vi "PropertyNodes.vi"() -> ()   [LabVIEW 2015]
panel:
  in  "stop":bool
  in  "Colors [4] 2":cluster{u32, u32}[](array[cluster])
  out "Colors [4]":cluster{u32, u32}[](array[cluster])
  in  "Legend:Visible":bool
  in  "Y Scale.Range:Maximum":dbl
  in  "Y Scale.Range:Minimum":dbl
  in  "X Scale.Range:Maximum":dbl
  in  "X Scale.Range:Minimum":dbl
  in  "Disabled 2":T1(ring)
  out "Waveform Chart":dbl(graph)
  in  "Numeric 2":dbl
  in  "Boolean 2":bool
  in  "Boolean":bool
  in  "Disabled":T1(ring)
  in  "Numeric":dbl
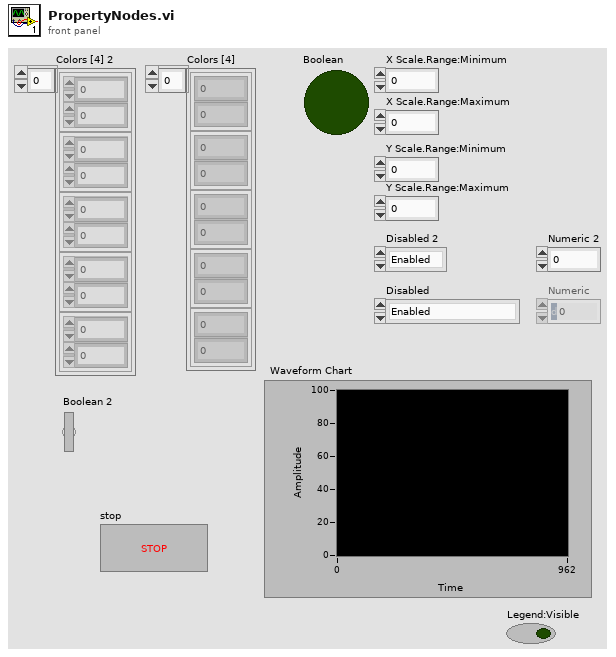
[diagram p1: front panel]
types:
  T1 = enum8{"Enabled", "Disabled", "Disabled and Grayed Out"}
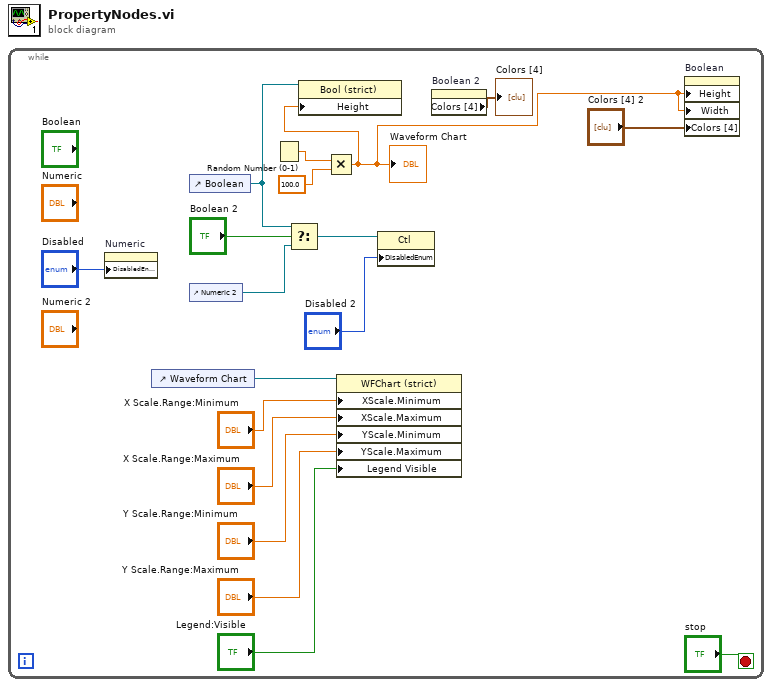
[diagram p0: block diagram]
diagram:
  n1 = while {
    stop <- "stop" stop-if-true
    n2 = property on="Numeric" class="DigNum (strict)"("DisabledEnum"="Disabled") -> ()  [unwired: 2 in, 2 out]
    n3 = control-ref of="Waveform Chart"() -> (w12:refnum<vi>)
    n4 = control-ref of="Boolean"() -> (w17:refnum<vi>)
    n5 = control-ref of="Numeric 2"() -> (w13:refnum<vi>)
    n6 = Random Number (0-1)() -> (number: 0 to 1=w14:dbl)
    n7 = Select(t=w17, s="Boolean 2", f=w13) -> (s? t:f=w2:refnum<vi>)
    n8 = Multiply(x=w14, y=100.0) -> (x*y=w4:dbl)
    "Waveform Chart" <- w4
    n9 = property class="Bool (strict)"(reference=w17, "Height"=w4) -> ()  [unwired: 1 in, 2 out]
    n10 = property class="WFChart (strict)"(reference=w12, "XScale.Minimum"="X Scale.Range:Minimum", "XScale.Maximum"="X Scale.Range:Maximum", "YScale.Minimum"="Y Scale.Range:Minimum", "YScale.Maximum"="Y Scale.Range:Maximum", "Legend Visible"="Legend:Visible") -> ()  [unwired: 1 in, 2 out]
    n11 = property class="Ctl"(reference=w2, "DisabledEnum"="Disabled 2") -> ()  [unwired: 1 in, 2 out]
    n12 = property on="Boolean 2" class="Bool (strict)"() -> ("Colors [4]"=→"Colors [4]":cluster{u32, u32}[])  [unwired: 2 in, 2 out]
    n13 = property on="Boolean" class="Bool (strict)"("Height"=w4, "Width"=w4, "Colors [4]"="Colors [4] 2") -> ()  [unwired: 2 in, 2 out]
  }
